vi "Error Check (SubVI).vi"(3 "calling VI":string="<<no text description>>", 4 "tag #":i32, 5 "error IN":errorcluster) -> (2 "error OUT":errorcluster)   [LabVIEW 2015]
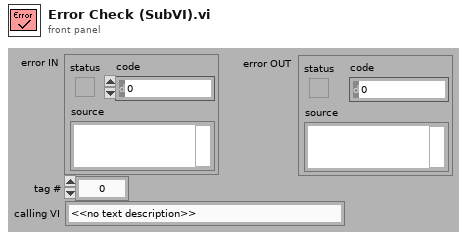
[diagram p1: front panel]
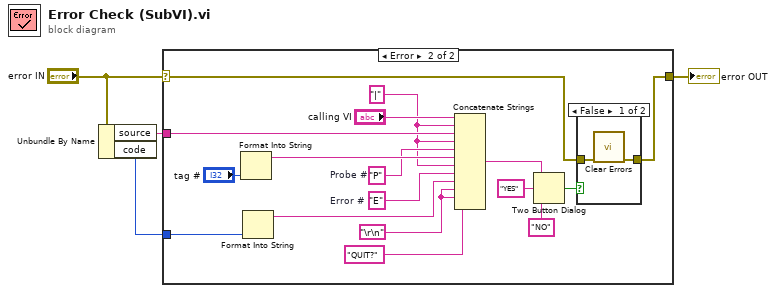
[diagram p0: block diagram]
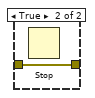
[diagram p3: hidden frame]
diagram:
  n1 = Unbundle By Name("error IN") -> ("source"=w4:string, "code"=w1:i32)
  n2 = case shown="Error" "error IN" {
    selector: "error IN" -> [w5 w8]
    tunnel: w4 -> [_ w22]
    tunnel: [w5 w7] -> w2
    tunnel: w1 -> [_ w19]
    frame No Error {
    }
    frame Error {
      w11 = "\r\n"
      w12 = "E"  # Error #
      w13 = "|" ("string")
      w14 = "P"  # Probe #
      n3 = Format Into String("tag #") -> (resulting string=w20:string)  [unwired: 3 in, 1 out]
      n4 = Format Into String(w19) -> (resulting string=w18:string)  [unwired: 3 in, 1 out]
      n5 = Concatenate Strings("calling VI", w13, w22, w13, w14, w20, w13, w12, w18, w11, w11, "QUIT?" ("message")) -> (w9:string)
      n6 = Two Button Dialog(message=w9, 1:"NO" ("F button name (\"Cancel\")"), 2:"YES" ("T button name (\"OK\")")) -> (T button?=w6:bool)
      n7 = case shown="False" w6 {
        tunnel: w8 -> [w24 w25]
        tunnel: [w23 w25] -> w7
        frame False {
          n8 = call <vilib>:"Clear Errors.vi"("error in (no error)"=w24) -> ("error out"=w23:errorcluster)  [unwired: 1 in, 5 out]
        }
        frame True {
          n9 = Stop() -> ()  [unwired: 1 out]
        }
      }
    }
  }
  "error OUT" <- w2
